vi "Test 01.vi"() -> ()   [LabVIEW 2021]
uses:
  <vilib>/Platform/TimedLoop/XDataNode/timing_clust.ctl
  <vilib>/Platform/TimedLoop/XDataNode/nitl_modes.ctl
  <vilib>/Platform/TimedLoop/XDataNode/wakeup.ctl
  <vilib>/MakerHub/LINX/Public/Utilities/Open Serial.vi
  <vilib>/Utility/file.llb/Write Delimited Spreadsheet (DBL).vi
  <vilib>/platform/TimedLoop/XDataNode/XDataNode.xnode
  <vilib>/Platform/TimedLoop/XDataNode/XDNodeRunTimeDep.lvlib
  <vilib>/MakerHub/LINX/LMH-LINX.lvlib
panel:
  out "dt":dbl
  out "Overrun":bool
  in  "Serial Port":refnum<visa-resource-name>
  in  "Stop Button":bool
  out "Angle":dbl(graph)=0.10008950000019468
  in  "Motor command":dbl
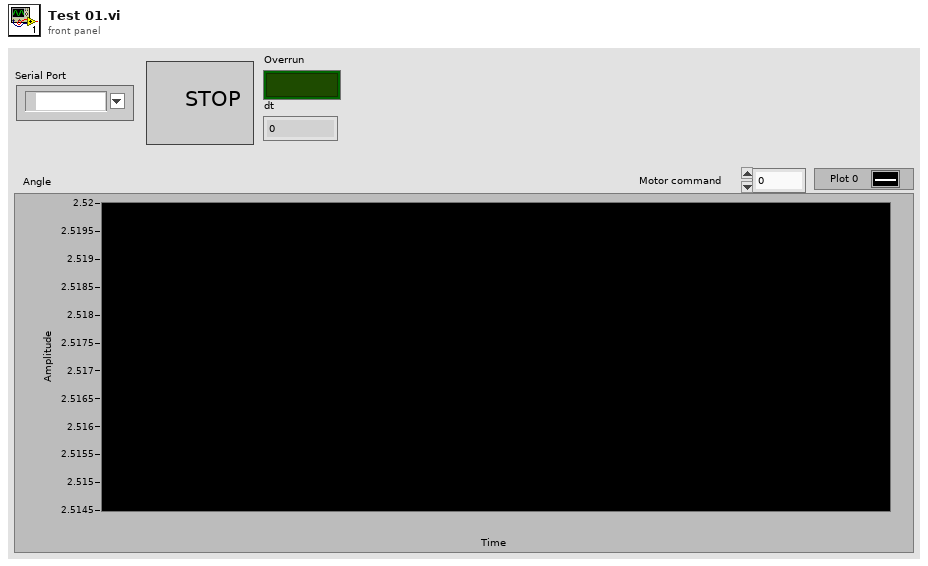
[diagram p1: front panel]
types:
  T1 = typedef "XDNodeRunTimeDep.lvlib/timing_clust.ctl" = cluster{"Expected End [f-1]":u64, "Actual End [f-1]":u64, "Finished Late? [f-1]":bool, "Expected End [i-1]":u64, "Actual End [i-1]":u64, "Finished Late? [i-1]":bool, "Expected Start [i]":u64, "Actual Start [i]":u64, "Expected Start [f]":u64, "Actual Start [f]":u64, "Source Name":string, "Structure Name":string, "Period":i64, "Deadline":i64, "Offset":i64, "Start":i64, "Priority":i32, "Timeout":i32, "Mode":T2, "Wakeup Reason":T3, "Error":errorcluster, "Source Type":string, "Secondary Source Type":string, "Global End Time":u64, "Global Start Time":u64, "Frame Duration":u64, "Iteration Duration":u64, "Assigned CPU":i32, "I/O Scan Engine Mode":u32}
  T2 = typedef "XDNodeRunTimeDep.lvlib/nitl_modes.ctl" = enum32{"No Change", "Process missed periods, maintain original phase", "Discard missed periods, maintain original phase", "Process missed periods, ignore original phase", "Discard missed periods, ignore original phase"}
  T3 = typedef "XDNodeRunTimeDep.lvlib/wakeup.ctl" = enum32{"Normal", "Aborted", "Asynchronous wakeup", "Timing source error", "Timed loop error", "Timeout"}
  T4 = typedef "LMH-LINX.lvlib/LINX Ref.ctl" = cluster{"IO":T5, "Interface":T6, "LINX Device Config":T7}
  T5 = typedef "LMH-LINX.lvlib/Platform.ctl" = enum16{"Remote", "Local"}
  T6 = typedef "LMH-LINX.lvlib/Interface.ctl" = enum16{"Serial", "TCP"}
  T7 = typedef "LMH-LINX.lvlib/Device.lvlib/LINX Device Config.ctl" = cluster{"Interface":T6, "COM Port":refnum<visa-resource-name>, "TCP Configuration":T8, "Device Family":u8, "Device ID":u8, "Device Name":string, "TCP Ref":refnum<k5>, "Channels":T9}
  T8 = typedef "LMH-LINX.lvlib/Device.lvlib/TCP Config.ctl" = cluster{"IP Address":string, "Port":u16}
  T9 = typedef "LMH-LINX.lvlib/Channels.ctl" = cluster{"DI":u8[], "DO":u8[], "AI":u8[], "AO":u8[], "PWM":u8[], "QE":u8[], "UART":u8[], "I2C 2":u8[], "SPI":u8[], "CAN":u8[], "Servo":u8[], "AI Ref (V)":dbl, "AI Resolution (Bits)":u8, "AO Ref (V)":dbl, "AO Resolution (Bits)":u8}
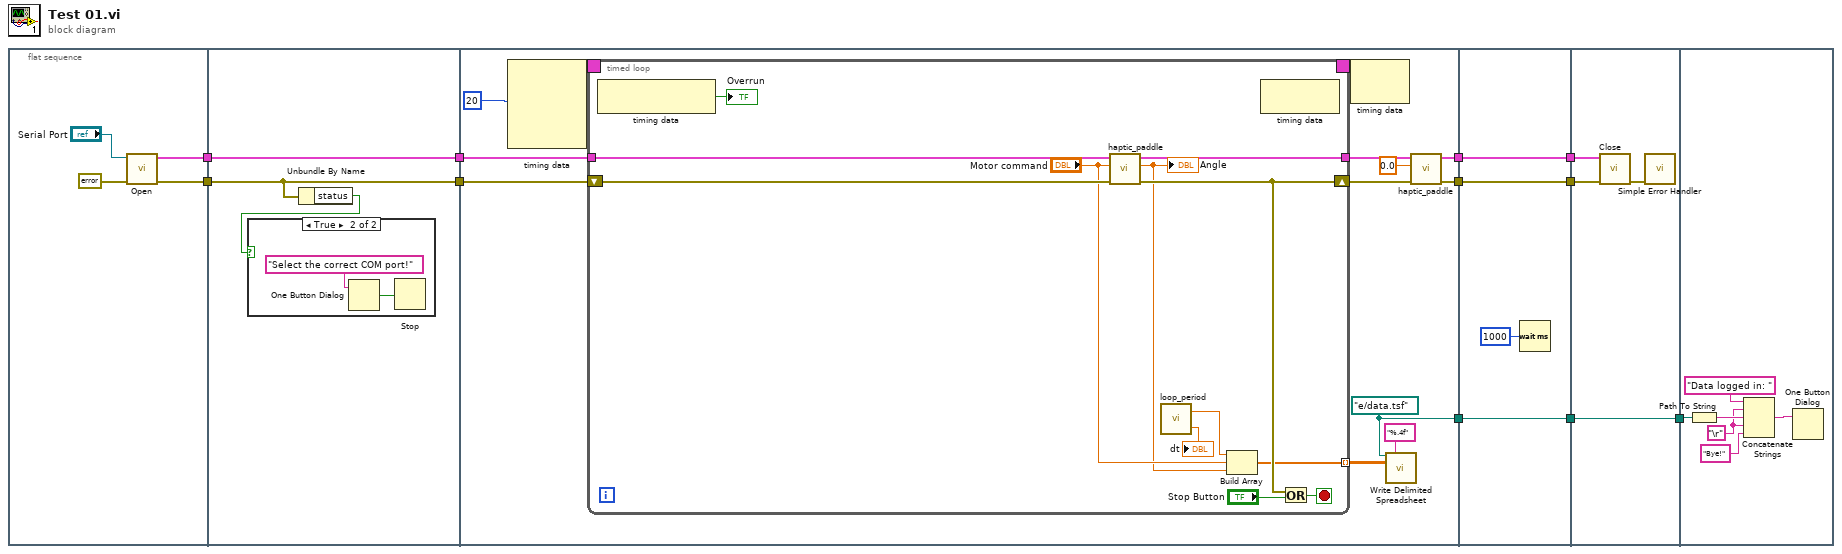
[diagram p0: block diagram]
diagram:
  n1 = flat-sequence {
    tunnel: [w13] -> w7
    tunnel: [w12] -> w5
    tunnel: w7 -> [w18]
    tunnel: [w18] -> w6
    tunnel: w5 -> [w17]
    tunnel: [w17] -> w4
    tunnel: [w28] -> w10
    tunnel: [w27] -> w8
    tunnel: w6 -> [w26]
    tunnel: w4 -> [w25]
    tunnel: [w21] -> w3
    tunnel: [w55] -> w11
    tunnel: w10 -> [w55]
    tunnel: [w54] -> w9
    tunnel: w8 -> [w54]
    tunnel: w3 -> [w53]
    tunnel: [w53] -> w2
    tunnel: w11 -> [w59]
    tunnel: w9 -> [w58]
    tunnel: w2 -> [w57]
    tunnel: [w57] -> w1
    tunnel: w1 -> [w66]
    frame #0 {
      n2 = call-poly <vilib>:"Open.vi"("Error In"=errorcluster {"status"=FALSE, "code"=0, "source"=""}, "Serial Port"="Serial Port") -> ("Error Out"=w12:errorcluster, "LINX Resource"=w13:T4)  [unwired: 7 in, 1 out]
    }
    frame #1 {
      n3 = Unbundle By Name(w17) -> ("status"=w16:bool)
      n4 = case shown="True" w16 {
        frame False {
        }
        frame True {
          n5 = One Button Dialog(message="Select the correct COM port!") -> (true=w19:bool)  [unwired: 1 in]
          n6 = Stop(stop? (T)=w19) -> ()
        }
      }
    }
    frame #2 {
      w21 = path "e:/data.tsf" ("file path (dialog if empty)")
      n7 = node-c288(i64 20 ("Period")) -> (w33:T1)  [unwired: 3 in]
      n8 = timed-loop {
        tunnel: w26 -> [w41]
        tunnel: [w43] -> w30
        shift-right: [w42] -> w29
        shift-left: w25 -> [w40]
        timing: w33 -> [_]
        timing-out: [_] -> w32
        tunnel: [w37] -> w23 mode=indexing
        stop <- w45 stop-if-true
        n9 = node-c288() -> (→"Overrun":bool)  [unwired: 1 in]
        n10 = call "haptic_paddle.vi"("Error In"=w40, "PWM Input"="Motor command", "LINX Resource In"=w41) -> ("Error Out"=w42:errorcluster, "Angular Output"=w38:dbl, "LINX Resource Out"=w43:T4)  [unwired: 6 in]
        "Angle" <- w38
        n11 = call "loop_period.vi"() -> ("dt"=→"dt":dbl, "t"=w36:dbl)  [unwired: 3 in]
        n12 = Build Array(w36, "Motor command", w38) -> (w37:dbl[])
        n13 = node-c288() -> ()  [unwired: 1 in, 1 out]
        n14 = Or(x=w42, y="Stop Button") -> (x .or. y?=w45:bool)
      }
      n15 = node-c288(w32) -> ()  [unwired: 1 out]
      n16 = call-poly <vilib>:"Write Delimited Spreadsheet.vi"("file path (dialog if empty)"=w21, "format (%.3f)"="%.4f", "2D data"=w23) -> ()  [unwired: 11 in, 2 out]
      n17 = call "haptic_paddle.vi"("Error In"=w29, "PWM Input"=0.0, "LINX Resource In"=w30) -> ("Error Out"=w27:errorcluster, "LINX Resource Out"=w28:T4)  [unwired: 6 in, 1 out]
    }
    frame #3 {
      n18 = Wait (ms)(milliseconds to wait=u32 1000) -> ()  [unwired: 1 out]
    }
    frame #4 {
      n19 = call <vilib>:"Close.vi"("Error In"=w58, "LINX Resource"=w59) -> ("Error Out"=w60:errorcluster)  [unwired: 9 in]
      n20 = call <vilib>:"Simple Error Handler.vi"("error in (no error)"=w60) -> ()  [unwired: 4 in, 5 out]
    }
    frame #5 {
      w61 = "\r"
      n21 = Path To String(path=w66) -> (string=w65:string)
      n22 = Concatenate Strings("Data logged in: " ("message"), w61, w65, w61, "Bye!" ("string")) -> (w63:string)
      n23 = One Button Dialog(message=w63) -> ()  [unwired: 1 in, 1 out]
    }
  }
